vi "detect modules.vi"(8 "error in":errorcluster, 10 "C Series module in":refnum<class "C Series Module.lvclass">, 11 "chassis in":refnum<class "Chassis.lvclass">) -> (0 "error out":errorcluster, 2 "C Series module out":refnum<class "C Series Module.lvclass">, 3 "chassis out":refnum<class "Chassis.lvclass">)   [LabVIEW 2014, in "SMI.lvlib" / "C Series Module.lvclass"]
uses:
  C Series Module.lvclass
  Chassis/Chassis.lvclass
  Device/read product name.vi
  Device/read device class.vi
  <vilib>/FPGAPlugInAG/Dynamic/niLvFpga_Close_Dynamic.vi
  <vilib>/regexp/Match Regular Expression.xnode
  <vilib>/rvi/interface/nirviCloseFPGA/nirviCloseFPGA.xnode
  Module/Module.lvclass
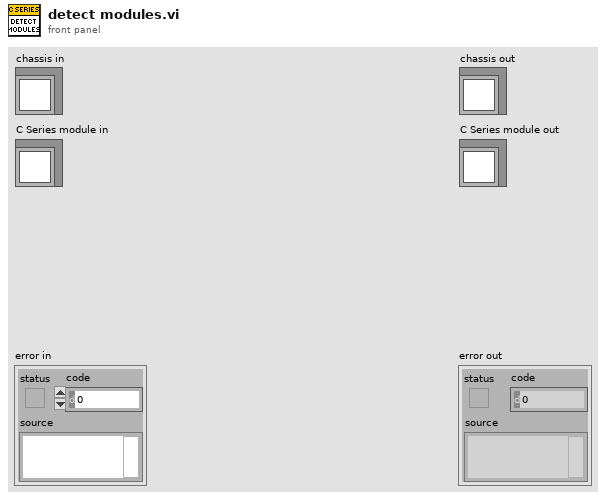
[diagram p1: front panel]
types:
  T1 = typedef "SMI.lvlib/Module.lvclass/module information.ctl" = cluster{"vendor name":string, "product name":string, "product ID":u16, "serial number":string}
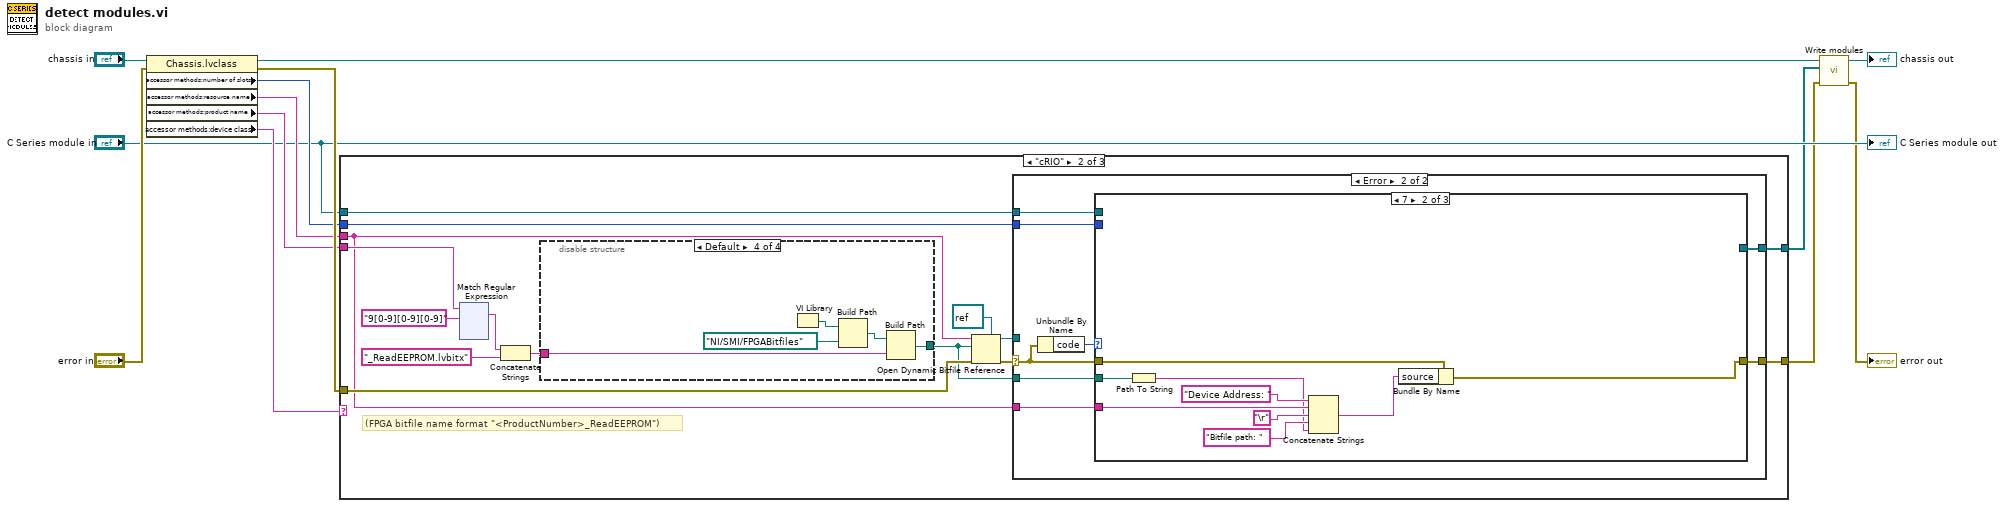
[diagram p0: block diagram]
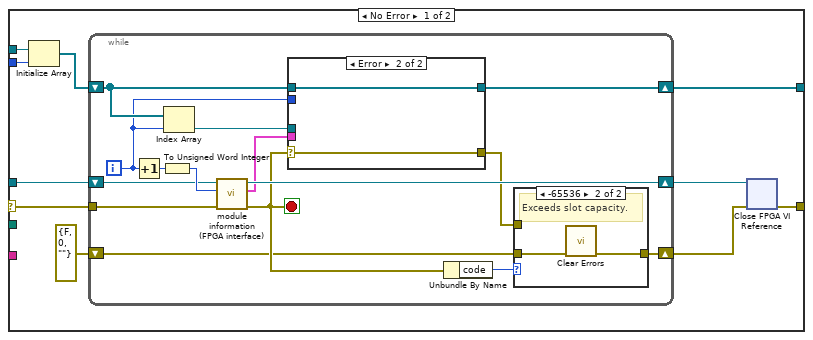
[diagram p3: hidden frame]
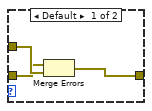
[diagram p4: hidden frame]
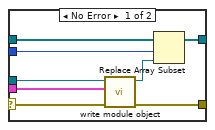
[diagram p5: hidden frame]
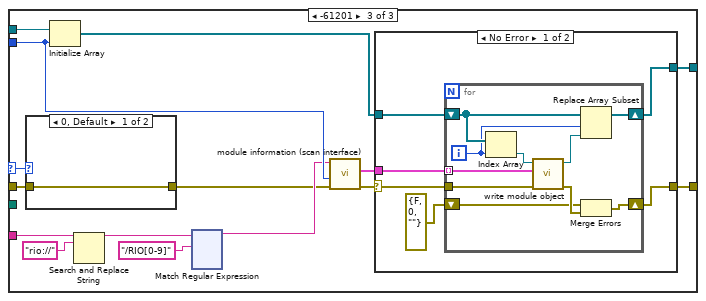
[diagram p7: hidden frame]
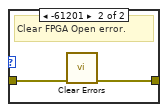
[diagram p9: hidden frame]
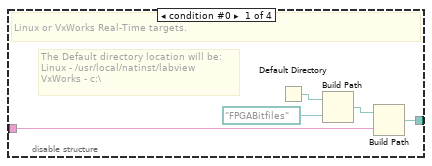
[diagram p10: hidden frame]
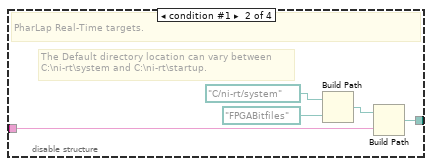
[diagram p11: hidden frame]
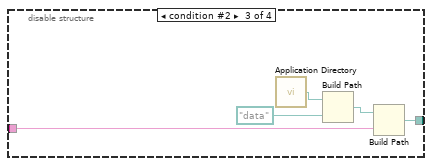
[diagram p12: hidden frame]
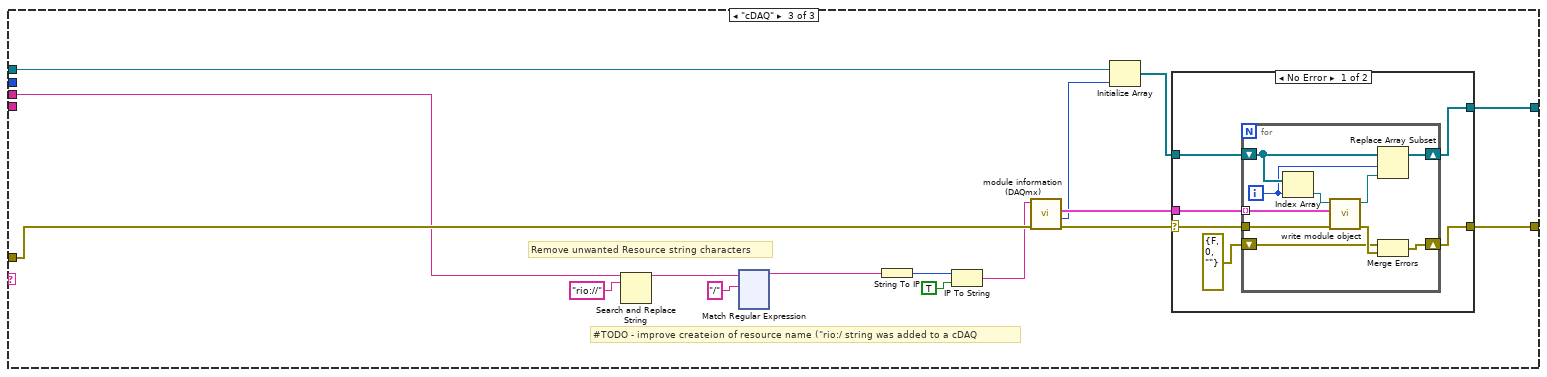
[diagram p13: hidden frame]
diagram:
  n1 = property class="Chassis.lvclass"(reference="chassis in", error in="error in") -> (reference out=w6:refnum<class "Chassis.lvclass">, error out=w12:errorcluster, "accessor methods:number of slots"=w7:i32, "accessor methods:resource name"=w8:string, "accessor methods:product name"=w9:string, "accessor methods:device class"=w10:string)
  n2 = case shown="\"cRIO\"" w10 {
    tunnel: [w14 w17 w383] -> w2
    tunnel: w12 -> [w14 w24 w386]
    tunnel: w9 -> [_ w29 _]
    tunnel: w8 -> [_ w16 w382]
    tunnel: w7 -> [_ w20 _]
    tunnel: "C Series module in" -> [_ w21 w385]
    tunnel: [_ w18 w384] -> w3
    frame Default {
      # "#TODO - Re-create block diagram (from lv2016 reference)."
    }
    frame "cRIO" {
      # "(FPGA bitfile name format \"<ProductNumber>_ReadEEPROM\")"
      n3 = xnode "Match Regular Expression"("input string"=w29, "regular expression"="9[0-9][0-9][0-9]") -> ("whole match"=w27:string)  [unwired: 4 in, 4 out]
      n4 = Concatenate Strings(w27, "_ReadEEPROM.lvbitx" ("string")) -> (w25:string)
      n5 = disable-structure shown="Default" {
        disable-tunnel: w25 -> [w238 w244 w249 w253]
        disable-tunnel: [w237 w243 w248 w252] -> w15
        frame condition #0 {
          # "The Default directory location will be:\nLinux - /usr/local/natinst/labview\nVxWorks - c:\\"
          # "Linux or VxWorks Real-Time targets."
          n6 = Default Directory() -> (w241:path)
          n7 = Build Path(base path=w241, name or relative path=path "FPGABitfiles") -> (appended path=w239:path)
          n8 = Build Path(base path=w239, name or relative path=w238) -> (appended path=w237:path)
        }
        frame condition #1 {
          # "The Default directory location can vary between\nC:\\ni-rt\\system and C:\\ni-rt\\startup."
          # "PharLap Real-Time targets."
          n9 = Build Path(base path=path "C:/ni-rt/system", name or relative path=path "FPGABitfiles") -> (appended path=w245:path)
          n10 = Build Path(base path=w245, name or relative path=w244) -> (appended path=w243:path)
        }
        frame condition #2 {
          n11 = call <vilib>:"Application Directory.vi"() -> ("Application Directory"=w247:path)
          n12 = Build Path(base path=w247, name or relative path=path "data") -> (appended path=w250:path)
          n13 = Build Path(base path=w250, name or relative path=w249) -> (appended path=w248:path)
        }
        frame condition #3 (active) {
          n14 = VI Library() -> (path=w256:path)
          n15 = Build Path(base path=w256, name or relative path=path "NI/SMI/FPGABitfiles") -> (appended path=w254:path)
          n16 = Build Path(base path=w254, name or relative path=w253) -> (appended path=w252:path)
        }
      }
      n17 = Open Dynamic Bitfile Reference(0:w16, 1:w15, 3:w24, 4:refnum<k20> refnum ("Refnum in")) -> (5:w22:refnum<k20>, 8:w23:errorcluster)  [unwired: 1 in]
      n18 = case shown="Error" w23 {
        selector: w23 -> [w36 w76]
        tunnel: w22 -> [w35 _]
        tunnel: w21 -> [w39 w75]
        tunnel: w20 -> [w38 w74]
        tunnel: [w34 w72] -> w18
        tunnel: [w30 w71] -> w17
        tunnel: w16 -> [_ w73]
        tunnel: w15 -> [_ w70]
        frame No Error {
          n19 = Initialize Array(w39, w38) -> (w37:refnum<class "C Series Module.lvclass">[])
          n20 = while {
            shift-right: [w46] -> w34
            shift-left: w37 -> [w47]
            tunnel: w36 -> [w54]
            shift-right: [w50] -> w32
            shift-left: w35 -> [w51]
            shift-right: [w40] -> w31
            shift-left: errorcluster {"status"=FALSE, "code"=0, "source"=""} ("error constant") -> [w41]
            i -> [w45]
            stop <- w44 stop-if-true
            n21 = Increment(x=w45) -> (x+1=w53:i32)
            n22 = To Unsigned Word Integer(number=w53) -> (unsigned 16bit integer=w52:u16)
            n23 = Index Array(array=w47, index=w45) -> (element=w49:refnum<class "C Series Module.lvclass">)
            n24 = call "module information (FPGA interface).vi"("error in"=w54, "Module"=w52, "Refnum in"=w51) -> ("error out"=w44:errorcluster, "Module Information"=w48:T1, "Refnum out"=w50:refnum<k20>)  [unwired: 6 in]
            n25 = case shown="Error" w44 {
              selector: w44 -> [w66 w68]
              tunnel: w49 -> [w67 _]
              tunnel: w48 -> [w65 _]
              tunnel: w47 -> [w64 w69]
              tunnel: [w63 w69] -> w46
              tunnel: w45 -> [w61 _]
              tunnel: [w60 w68] -> w42
              frame No Error {
                n26 = call "write module object.vi"("error in"=w66, "module information"=w65, "Module in"=w67) -> ("error out"=w60:errorcluster, "Module out"=w62:refnum<class "C Series Module.lvclass">)  [unwired: 7 in]
                n27 = Replace Array Subset(array=w64, new element=w62, index=w61) -> (w63:refnum<class "C Series Module.lvclass">[])
              }
              frame Error {
              }
            }
            n28 = Unbundle By Name(w44) -> ("code"=w43:i32)
            n29 = case shown="-65536" w43 {
              tunnel: w42 -> [w57 _]
              tunnel: w41 -> [w56 w59]
              tunnel: [w55 w58] -> w40
              frame Default {
                n30 = Merge Errors(w56, w57) -> (w55:errorcluster)
              }
              frame -65536 {
                # "Exceeds slot capacity."
                n31 = call <vilib>:"Clear Errors.vi"("error in (no error)"=w59) -> ("error out"=w58:errorcluster)  [unwired: 5 in, 1 out]
              }
            }
          }
          n32 = xnode "Close FPGA VI Reference"("FPGA VI Reference In"=w32, "error in"=w31) -> ("error out"=w30:errorcluster)
        }
        frame Error {
          n33 = Unbundle By Name(w76) -> ("code"=w77:i32)
          n34 = case shown="7" w77 {
            selector: w77 -> [_ _ w102]
            tunnel: w76 -> [w78 w81 w101]
            tunnel: w75 -> [_ _ w100]
            tunnel: w74 -> [_ _ w99]
            tunnel: w73 -> [_ w84 w94]
            tunnel: [_ _ w89] -> w72
            tunnel: [w78 w79 w88] -> w71
            tunnel: w70 -> [_ w83 _]
            frame Default {
            }
            frame 7 {
              n35 = Path To String(path=w83) -> (string=w82:string)
              n36 = Concatenate Strings("Device Address: ", w84, "\r", "Bitfile path: ", w82) -> (w80:string)
              n37 = Bundle By Name(cluster=w81, "source"=w80) -> (w79:errorcluster)
            }
            frame -61201 {
              n38 = case shown="0, Default" w102 {
                tunnel: w101 -> [w234 w236]
                tunnel: [w234 w235] -> w95
                frame 0, Default {
                }
                frame -61201 {
                  # "Clear FPGA Open error."
                  n39 = call <vilib>:"Clear Errors.vi"("error in (no error)"=w236) -> ("error out"=w235:errorcluster)  [unwired: 5 in, 1 out]
                }
              }
              n40 = Initialize Array(w100, w99) -> (w90:refnum<class "C Series Module.lvclass">[])
              n41 = Search and Replace String(input string=w94, search string="rio://") -> (result string=w92:string)  [unwired: 6 in, 3 out]
              n42 = xnode "Match Regular Expression"("input string"=w92, "regular expression"="/RIO[0-9]") -> ("before match"=w96:string)  [unwired: 4 in, 4 out]
              n43 = call "module information (scan interface).vi"("error in"=w95, "number of slots"=w99, "IP address (localhost)"=w96) -> ("error out"=w98:errorcluster, "module information"=w97:T1[])  [unwired: 7 in]
              n44 = case shown="No Error" w98 {
                selector: w98 -> [w219 w233]
                tunnel: w97 -> [w222 _]
                tunnel: w90 -> [w221 _]
                tunnel: [w218 _] -> w89
                tunnel: [w217 w233] -> w88
                frame No Error {
                  n45 = for {
                    tunnel: w222 -> [w232] mode=indexing
                    shift-right: [w225] -> w218
                    shift-left: w221 -> [w226]
                    shift-right: [w227] -> w217
                    shift-left: errorcluster {"status"=FALSE, "code"=0, "source"=""} ("error constant") -> [w229]
                    tunnel: w219 -> [w231]
                    i -> [w224]
                    n46 = Index Array(array=w226, index=w224) -> (element=w228:refnum<class "C Series Module.lvclass">)
                    n47 = call "write module object.vi"("error in"=w231, "module information"=w232, "Module in"=w228) -> ("error out"=w230:errorcluster, "Module out"=w223:refnum<class "C Series Module.lvclass">)  [unwired: 7 in]
                    n48 = Replace Array Subset(array=w226, new element=w223, index=w224) -> (w225:refnum<class "C Series Module.lvclass">[])
                    n49 = Merge Errors(w229, w230) -> (w227:errorcluster)
                  }
                }
                frame Error {
                }
              }
            }
          }
        }
      }
    }
    frame "cDAQ" {
      # "#TODO - improve createion of resource name (\"rio:/ string was added to a cDAQ"
      # "Remove unwanted Resource string characters"
      n50 = Search and Replace String(input string=w382, search string="rio://") -> (result string=w378:string)  [unwired: 6 in, 3 out]
      n51 = xnode "Match Regular Expression"("input string"=w378, "regular expression"="/") -> ("before match"=w374:string)  [unwired: 4 in, 4 out]
      n52 = String To IP(1:w374) -> (0:w373:u32)
      n53 = IP To String(1:TRUE ("dot notation? (F)"), 2:w373) -> (0:w371:string)
      n54 = call "module information (DAQmx).vi"("error in"=w386, "IP address (localhost)"=w371) -> ("error out"=w381:errorcluster, "number of slots"=w375:i32, "module information"=w380:T1[])  [unwired: 7 in]
      n55 = Initialize Array(w385, w375) -> (w376:refnum<class "C Series Module.lvclass">[])
      n56 = case shown="No Error" w381 {
        selector: w381 -> [w503 w517]
        tunnel: w380 -> [w506 _]
        tunnel: w376 -> [w505 _]
        tunnel: [w502 _] -> w384
        tunnel: [w501 w517] -> w383
        frame No Error {
          n57 = for {
            tunnel: w506 -> [w516] mode=indexing
            shift-right: [w509] -> w502
            shift-left: w505 -> [w510]
            shift-right: [w511] -> w501
            shift-left: errorcluster {"status"=FALSE, "code"=0, "source"=""} ("error constant") -> [w513]
            tunnel: w503 -> [w515]
            i -> [w508]
            n58 = Index Array(array=w510, index=w508) -> (element=w512:refnum<class "C Series Module.lvclass">)
            n59 = call "write module object.vi"("error in"=w515, "module information"=w516, "Module in"=w512) -> ("error out"=w514:errorcluster, "Module out"=w507:refnum<class "C Series Module.lvclass">)  [unwired: 7 in]
            n60 = Replace Array Subset(array=w510, new element=w507, index=w508) -> (w509:refnum<class "C Series Module.lvclass">[])
            n61 = Merge Errors(w513, w514) -> (w511:errorcluster)
          }
        }
        frame Error {
        }
      }
    }
  }
  n62 = call-dynamic "Write modules.vi"("error in (no error)"=w2, "modules"=w3, "Chassis in"=w6) -> ("error out"=→"error out":errorcluster, "Chassis out"=→"chassis out":refnum<class "Chassis.lvclass">)  [unwired: 7 in]
  "C Series module out" <- "C Series module in"
